vi "Get Enqueuer.vi"(8 "error in":errorcluster, 10 "Ident":string, 11 "Panel Actor Template in":refnum<class "Network Management UI.lvclass">) -> (0 "error out":errorcluster, 2 "Nested Enqueuer":refnum<class "Message Enqueuer.lvclass">, 3 "Panel Actor Template out":refnum<class "Network Management UI.lvclass">)   [LabVIEW 2020, in "Network Management UI.lvlib" / "Network Management UI.lvclass"]
uses:
  Network Management UI.lvclass
  Network Management UI.lvclass/Network Management UI.ctl
  <vilib>/ActorFramework/Message Enqueuer/Message Enqueuer.lvclass
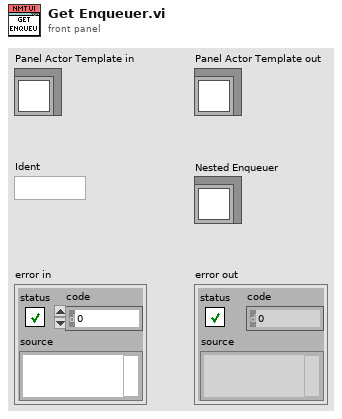
[diagram p1: front panel]
types:
  T1 = map{string, refnum<class "Message Enqueuer.lvclass">}
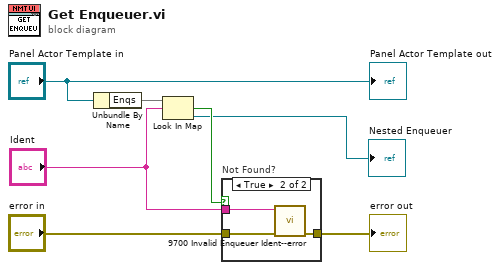
[diagram p0: block diagram]
diagram:
  n1 = Unbundle By Name("Panel Actor Template in") -> ("Enqs"=w6:T1)
  n2 = Look In Map(map=w6, key="Ident") -> (key not found?=w5:bool, value=→"Nested Enqueuer":refnum<class "Message Enqueuer.lvclass">)  [unwired: 1 in]
  n3 = case "Not Found?" shown="True" w5 {
    tunnel: "error in" -> [w8 w11]
    tunnel: [w8 w10] -> w3
    tunnel: "Ident" -> [_ w9]
    frame False {
    }
    frame True {
      n4 = call "9700 Invalid Enqueuer Ident--error.vi"("error in"=w11, "Ident"=w9) -> ("error out"=w10:errorcluster)  [unwired: 9 in]
    }
  }
  "error out" <- w3
  "Panel Actor Template out" <- "Panel Actor Template in"
